vi "Get Joystick 2017.vi"() -> (3 "Pilot-CoPilot Controls":T1)   [LabVIEW 2016]
uses:
  Robot Control Outputs 2017.ctl
  Global Variables/Refnum Names.vi
  <vilib>/Rock Robotics/WPI/Utilities/WPI_GetSetVariantRefNum.vi
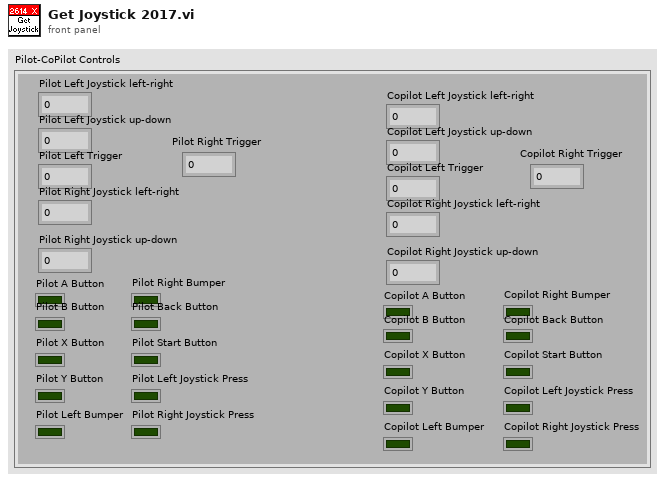
[diagram p1: front panel]
types:
  T1 = typedef "Robot Control Outputs 2017.ctl" = cluster{"Pilot Left Joystick left-right":dbl, "Pilot Left Joystick up-down":dbl, "Pilot A Button":bool, "Pilot B Button":bool, "Pilot X Button":bool, "Pilot Y Button":bool, "Pilot Left Bumper":bool, "Pilot Right Bumper":bool, "Pilot Back Button":bool, "Pilot Start Button":bool, "Pilot Left Joystick Press":bool, "Pilot Right Joystick Press":bool, "Pilot Left Trigger":dbl, "Pilot Right Joystick left-right":dbl, "Pilot Right Joystick up-down":dbl, "Pilot Right Trigger":dbl, "Copilot Left Joystick left-right":dbl, "Copilot Left Joystick up-down":dbl, "Copilot A Button":bool, "Copilot B Button":bool, "Copilot X Button":bool, "Copilot Y Button":bool, "Copilot Left Bumper":bool, "Copilot Right Bumper":bool, "Copilot Back Button":bool, "Copilot Start Button":bool, "Copilot Left Joystick Press":bool, "Copilot Right Joystick Press":bool, "Copilot Left Trigger":dbl, "Copilot Right Joystick left-right":dbl, "Copilot Right Joystick up-down":dbl, "Copilot Right Trigger":dbl}
  T2 = typedef "WPI_JoystickDevRef.ctl" = cluster{"Device":T3}
  T3 = typedef "WPI_JoystickDeviceEnum.ctl" = enum16{"USB 0", "USB 1", "USB 2", "USB 3", "USB 4", "USB 5"}
  T4 = cluster{"Axes[0]":dbl, "Axes[1]":dbl, "Axes[2]":dbl, "Axes[3]":dbl, "Axes[4]":dbl, "Axes[5]":dbl, "Axes[6]":dbl, "Axes[7]":dbl, "Axes[8]":dbl}
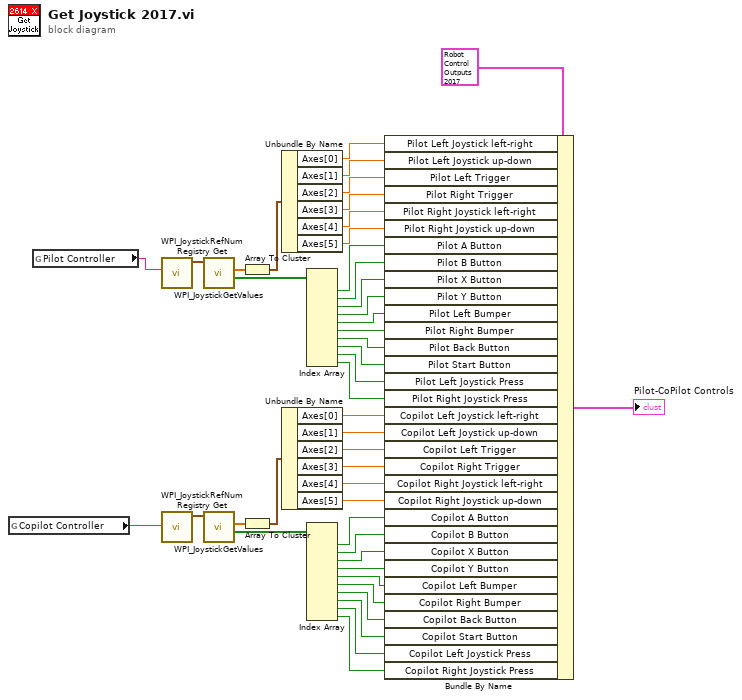
[diagram p0: block diagram]
diagram:
  n1 = global read "Refnum Names.vi" "Copilot Controller"() -> (w2:string)
  n2 = global read "Refnum Names.vi" "Pilot Controller"() -> (w1:string)
  n3 = call <vilib>:"WPI_JoystickRefNum Registry Get.vi"("refnum name"=w1) -> ("JoystickDevRef"=w44:T2)  [unwired: 9 in, 1 out]
  n4 = call <vilib>:"WPI_JoystickRefNum Registry Get.vi"("refnum name"=w2) -> ("JoystickDevRef"=w24:T2)  [unwired: 9 in, 1 out]
  n5 = call <vilib>:"WPI_JoystickGetValues.vi"("JoystickDevRef"=w44) -> ("Buttons"=w35:bool[], "Axes"=w43:dbl[])  [unwired: 6 in, 3 out]
  n6 = call <vilib>:"WPI_JoystickGetValues.vi"("JoystickDevRef"=w24) -> ("Buttons"=w22:bool[], "Axes"=w23:dbl[])  [unwired: 6 in, 3 out]
  n7 = Array To Cluster(array=w43) -> (cluster=w42:T4)
  n8 = Array To Cluster(array=w23) -> (cluster=w21:T4)
  n9 = Unbundle By Name(w42) -> ("Axes[0]"=w41:dbl, "Axes[1]"=w40:dbl, "Axes[2]"=w39:dbl, "Axes[3]"=w38:dbl, "Axes[4]"=w37:dbl, "Axes[5]"=w36:dbl)
  n10 = Unbundle By Name(w21) -> ("Axes[0]"=w20:dbl, "Axes[1]"=w19:dbl, "Axes[2]"=w18:dbl, "Axes[3]"=w17:dbl, "Axes[4]"=w16:dbl, "Axes[5]"=w15:dbl)
  n11 = Index Array(array=w35) -> (element #1=w34:bool, element #2=w33:bool, element #3=w32:bool, element #4=w31:bool, element #5=w30:bool, element #6=w29:bool, element #7=w28:bool, element #8=w27:bool, element #9=w26:bool, element #10=w25:bool)  [unwired: 10 in]
  n12 = Index Array(array=w22) -> (element #1=w14:bool, element #2=w13:bool, element #3=w12:bool, element #4=w11:bool, element #5=w9:bool, element #6=w10:bool, element #7=w8:bool, element #8=w7:bool, element #9=w6:bool, element #10=w5:bool)  [unwired: 10 in]
  n13 = Bundle By Name(cluster=T1 {"Pilot Left Joystick left-right"=0.0, "Pilot Left Joystick up-down"=0.0, "Pilot A Button"=FALSE, "Pilot B Button"=FALSE, "Pilot X Button"=FALSE, "Pilot Y Button"=FALSE, "Pilot Left Bumper"=FALSE, "Pilot Right Bumper"=FALSE, "Pilot Back Button"=FALSE, "Pilot Start Button"=FALSE, "Pilot Left Joystick Press"=FALSE, "Pilot Right Joystick Press"=FALSE, "Pilot Left Trigger"=0.0, "Pilot Right Joystick left-right"=0.0, "Pilot Right Joystick up-down"=0.0, "Pilot Right Trigger"=0.0, "Copilot Left Joystick left-right"=0.0, "Copilot Left Joystick up-down"=0.0, "Copilot A Button"=FALSE, "Copilot B Button"=FALSE, "Copilot X Button"=FALSE, "Copilot Y Button"=FALSE, "Copilot Left Bumper"=FALSE, "Copilot Right Bumper"=FALSE, "Copilot Back Button"=FALSE, "Copilot Start Button"=FALSE, "Copilot Left Joystick Press"=FALSE, "Copilot Right Joystick Press"=FALSE, "Copilot Left Trigger"=0.0, "Copilot Right Joystick left-right"=0.0, "Copilot Right Joystick up-down"=0.0, "Copilot Right Trigger"=0.0} ("Pilot-CoPilot Controls"), "Pilot Left Joystick left-right"=w41, "Pilot Left Joystick up-down"=w40, "Pilot Left Trigger"=w39, "Pilot Right Trigger"=w38, "Pilot Right Joystick left-right"=w37, "Pilot Right Joystick up-down"=w36, "Pilot A Button"=w34, "Pilot B Button"=w33, "Pilot X Button"=w32, "Pilot Y Button"=w31, "Pilot Left Bumper"=w30, "Pilot Right Bumper"=w29, "Pilot Back Button"=w28, "Pilot Start Button"=w27, "Pilot Left Joystick Press"=w26, "Pilot Right Joystick Press"=w25, "Copilot Left Joystick left-right"=w20, "Copilot Left Joystick up-down"=w19, "Copilot Left Trigger"=w18, "Copilot Right Trigger"=w17, "Copilot Right Joystick left-right"=w16, "Copilot Right Joystick up-down"=w15, "Copilot A Button"=w14, "Copilot B Button"=w13, "Copilot X Button"=w12, "Copilot Y Button"=w11, "Copilot Left Bumper"=w9, "Copilot Right Bumper"=w10, "Copilot Back Button"=w8, "Copilot Start Button"=w7, "Copilot Left Joystick Press"=w6, "Copilot Right Joystick Press"=w5) -> (→"Pilot-CoPilot Controls":T1)
